vi "Launch Tree Load.vi"(11 "QControlWizard in":refnum<class "QControl Creation Wizard.lvclass">) -> (0 "error out":errorcluster, 3 "QControlWizard out":refnum<class "QControl Creation Wizard.lvclass">)   [LabVIEW 2015, in "QControl Creation Wizard.lvclass"]
uses:
  QControl Creation Wizard.lvclass
  QControl Creation Wizard.lvclass/QControl Creation Wizard.ctl
  New QControl Info/New QControl Info.lvclass/New QControl Info.ctl
  New QControl Info/Read App Refnum.vi
  Async Tree Load.vi
  QControl Classes/TreeSelectionSingle/TreeSelectionSingle.lvclass
  New QControl Info/New QControl Info.lvclass
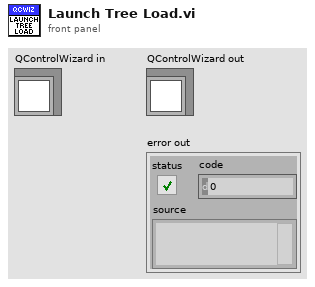
[diagram p1: front panel]
types:
  T1 = enum8{"Enabled", "Disabled", "Disabled and Grayed Out"}
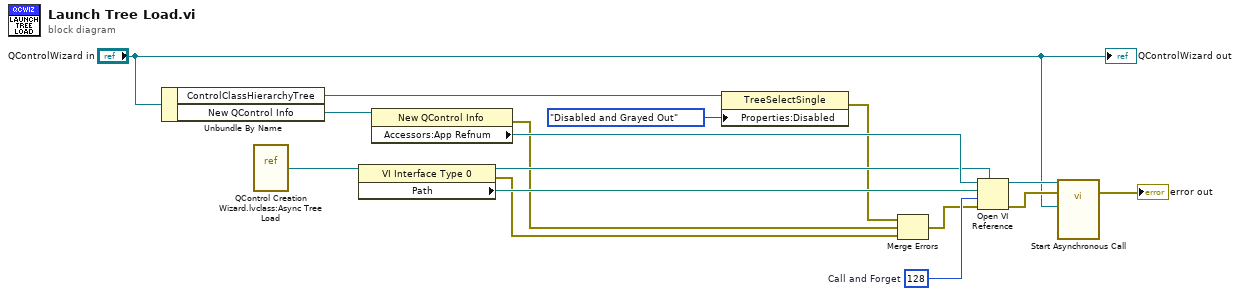
[diagram p0: block diagram]
diagram:
  w12 = 128  # Call and Forget
  n1 = Unbundle By Name("QControlWizard in") -> ("ControlClassHierarchyTree"=w3:refnum<class "TreeSelectionSingle.lvclass">, "New QControl Info"=w16:refnum<data-value>)
  n2 = vi-ref "QControl Creation Wizard.lvclass:Async Tree Load.vi"() -> (w14:refnum<vi>)
  n3 = property class="VI Interface Type 0"(reference=w14) -> (reference out=w11:refnum<vi>, error out=w10:errorcluster, "Path"=w15:path)  [unwired: 1 in]
  n4 = property class="New QControl Info"(reference=w16) -> (error out=w8:errorcluster, "Accessors:App Refnum"=w13:refnum<vi>)  [unwired: 1 in, 1 out]
  n5 = property class="TreeSelectSingle"(reference=w3, "Properties:Disabled"=T1."Disabled and Grayed Out" ("Disabled")) -> (error out=w1:errorcluster)  [unwired: 1 in, 1 out]
  n6 = Merge Errors(w1, w8, w10) -> (w9:errorcluster)
  n7 = Open VI Reference(type specifier VI Refnum (for type only)=w11, application reference (local)=w13, vi path=w15, options=w12, error in (no error)=w9) -> (vi reference=w7:refnum<vi>, error out=w6:errorcluster)  [unwired: 1 in]
  n8 = call-by-ref "Start Asynchronous Call"(reference=w7, error in=w6, "QControlWizard in"="QControlWizard in") -> (error out=→"error out":errorcluster)  [unwired: 10 in, 2 out]
  "QControlWizard out" <- "QControlWizard in"
